vi "Parse URI.vi"(0 "URI":string="ws://hostname.domain:80/resource/name", 7 "URI type (WS)":enum16{"WS", "HTTP"}(ring), 11 "error in":errorcluster) -> (4 "URI Out":string="ws://hostname.domain:80/resource/name", 6 "Hostname":string, 8 "HTTP URI":string, 10 "Resource Name":string, 13 "Port":u16, 14 "Default Port":bool, 15 "error out":errorcluster)   [LabVIEW 2016, in "WebSockets.lvlib"]
doc: "Parses a websocket or HTTP URI and outputs its components"
uses:
  WebSockets.lvlib
  <vilib>/Utility/error.llb/Error Cluster From Error Code.vi
  <vilib>/regexp/Match Regular Expression.xnode
  <vilib>/ErrorRing/Error Ring.xnode
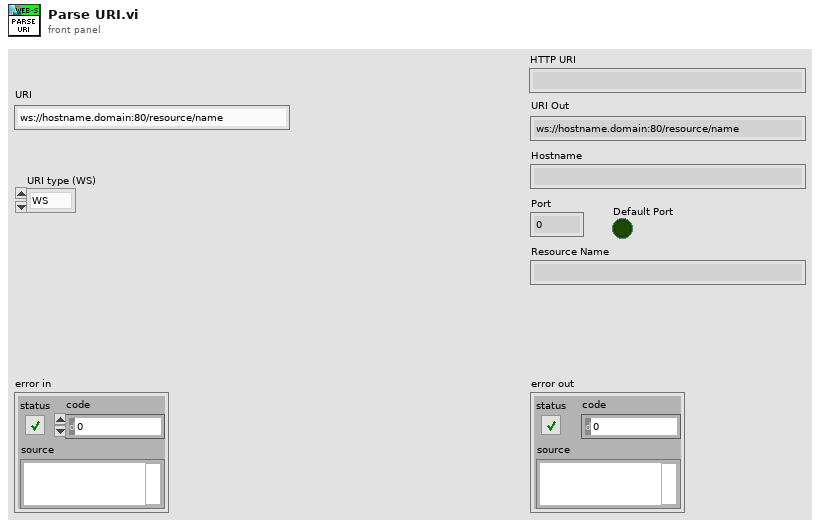
[diagram p1: front panel]
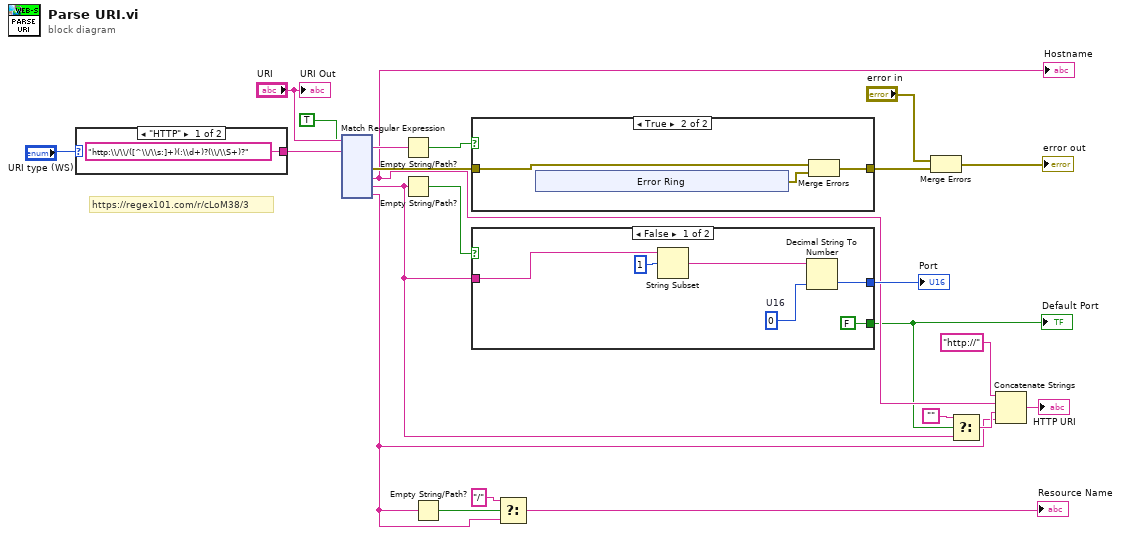
[diagram p0: block diagram]
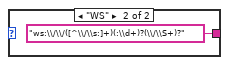
[diagram p2: hidden frame]
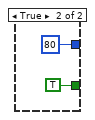
[diagram p4: hidden frame]
diagram:
  # "https://regex101.com/r/cLoM38/3"
  n1 = case shown="\"HTTP\"" "URI type (WS)" {
    tunnel: ["http:\\/\\/([^\\/\\s:]+)(:\\d+)?(\\/\\S+)?" ("regular expression") "ws:\\/\\/([^\\/\\s:]+)(:\\d+)?(\\/\\S+)?" ("regular expression")] -> w22
    frame "HTTP" {
    }
    frame "WS" {
    }
  }
  n2 = xnode "Match Regular Expression"("input string"="URI", "regular expression"=w22, "ignore case? (F)"=TRUE) -> ("whole match"=w18:string, "error out"=w15:errorcluster, "submatch 1"=w8:string, "submatch 2"=w6:string, "submatch 3"=w3:string)  [unwired: 3 in, 3 out]
  "Hostname" <- w8
  n3 = Empty String/Path?(string/path=w18) -> (empty?=w16:bool)
  n4 = Empty String/Path?(string/path=w6) -> (empty?=w21:bool)
  n5 = Empty String/Path?(string/path=w3) -> (empty?=w12:bool)
  n6 = case shown="True" w16 {
    tunnel: w15 -> [w26 w29]
    tunnel: [w26 w27] -> w14
    frame False {
    }
    frame True {
      n7 = xnode ("Error Ring")() -> ("error out"=w28:errorcluster)
      n8 = Merge Errors(w29, w28) -> (w27:errorcluster)
    }
  }
  n9 = case shown="False" w21 {
    tunnel: w6 -> [w37 _]
    tunnel: [w36 u16 80] -> w20
    tunnel: [FALSE TRUE] -> w7
    frame False {
      w38 = u16 0  # U16
      n10 = String Subset(string=w37, offset (0)=1) -> (substring=w39:string)  [unwired: 1 in]
      n11 = Decimal String To Number(string=w39, default (0L)=w38) -> (number=w36:u16)  [unwired: 1 in, 1 out]
    }
    frame True {
    }
  }
  "Default Port" <- w7
  "Port" <- w20
  n12 = Select(t="/", s=w12, f=w3) -> (s? t:f=→"Resource Name":string)
  n13 = Merge Errors("error in", w14) -> (→"error out":errorcluster)
  n14 = Select(t="", s=w7, f=w6) -> (s? t:f=w4:string)
  n15 = Concatenate Strings("http://" ("string"), w8, w4, w3) -> (→"HTTP URI":string)
  "URI Out" <- "URI"
